vi "判断判别式.vi"(7 "A":dbl, 10 "C":dbl, 11 "B":dbl) -> (3 "判别式是否大于等于0":bool)   [LabVIEW 2018]
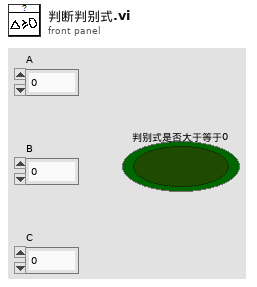
[diagram p1: front panel]
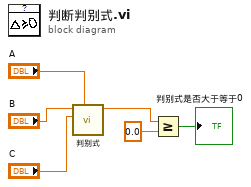
[diagram p0: block diagram]
diagram:
  n1 = call "判别式.vi"("A"="A", "C"="C", "B"="B") -> ("判别式"=w1:dbl)  [unwired: 8 in]
  n2 = Greater Or Equal?(x=w1, y=0.0) -> (x >= y?=→"判别式是否大于等于0":bool)
